vi "Get Fullscale.vi"(8 "Error In (no error)":errorcluster, 11 "VISA Resource Name":refnum<visa-resource-name>) -> (0 "Error Out":errorcluster, 2 "Full Scale":dbl format="%.5f", 3 "VISA Resource Name Out":refnum<visa-resource-name>)   [LabVIEW 2010, in "Stanford Research 844.lvlib"]
doc: "This VI queries for full scale mode."
uses:
  <instrlib>/Stanford Research 844/Stanford Research 844.lvlib
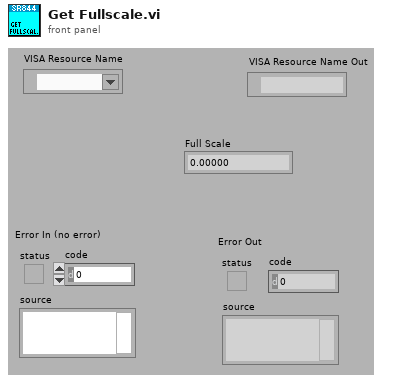
[diagram p1: front panel]
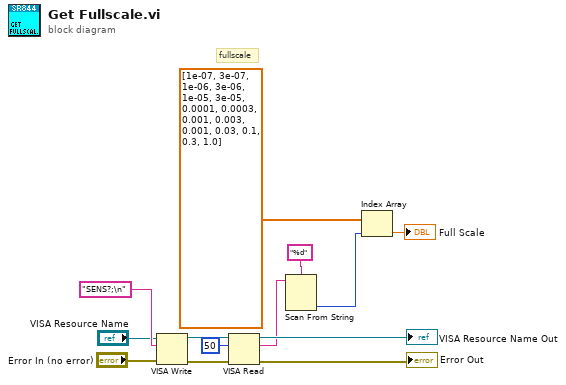
[diagram p0: block diagram]
diagram:
  # "fullscale"
  n1 = VISA Write(VISA resource name="VISA Resource Name", write buffer="SENS?;\n" ("write buffer (\"\")"), error in (no error)="Error In (no error)") -> (VISA resource name out=w12:refnum<visa-resource-name>, error out=w11:errorcluster)  [unwired: 1 out]
  n2 = VISA Read(VISA resource name=w12, byte count=u32 50 ("byte count (0)"), error in (no error)=w11) -> (VISA resource name out=→"VISA Resource Name Out":refnum<visa-resource-name>, read buffer=w7:string, error out=→"Error Out":errorcluster)  [unwired: 1 out]
  n3 = Scan From String(format string="%d", input string=w7) -> (output 1=w3:i32)  [unwired: 3 in, 3 out]
  n4 = Index Array(array=dbl[] [1e-07, 3e-07, 1e-06, 3e-06, 1e-05, 3e-05, 0.0001, 0.0003, 0.001, 0.003, 0.001, 0.03, 0.1, 0.3, 1.0], index=w3) -> (element=→"Full Scale":dbl)
